vi "Get Result.vi"(6 "Last request":bool, 8 "error in (no error)":errorcluster, 11 "Temperature Controller Driver in":refnum<class "Temperature Controller Driver.lvclass">) -> (0 "error out":errorcluster, 2 "Result":refnum<class "Acquired Result.lvclass">, 3 "Temperature Controller Driver out":refnum<class "Temperature Controller Driver.lvclass">)   [LabVIEW 2024, in "Temperature Controller Driver.lvclass"]
uses:
  Temperature Controller Driver.lvclass
  Results/Acquired Result/Acquired Result.lvclass
  Temperature Controller Driver.lvclass/Temperature Controller Driver.ctl
  d4704567-7086-47cf-bd59-7ca7029b5dc6.vi
  28732cff-cc5e-42dd-a4af-5e59016cd5d7.vi
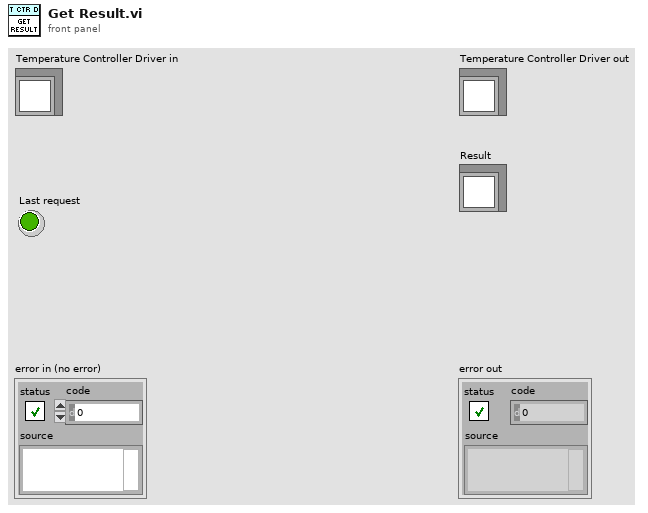
[diagram p1: front panel]
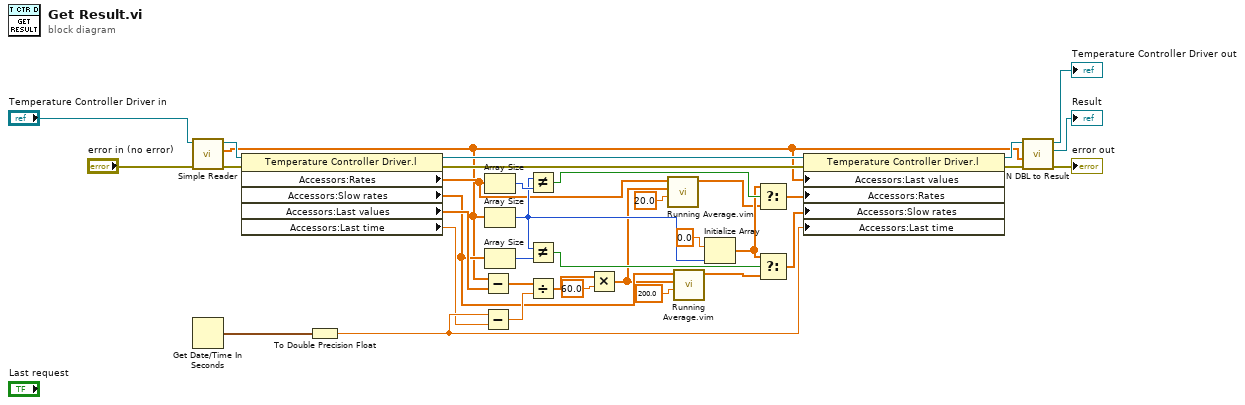
[diagram p0: block diagram]
diagram:
  n1 = call-dynamic "Simple Reader.vi"("error in (no error)"="error in (no error)", "Instrument Driver in"="Temperature Controller Driver in") -> ("error out"=w36:errorcluster, "Signals"=w4:dbl[], "Instrument Driver out"=w30:refnum<class "Temperature Controller Driver.lvclass">)  [unwired: 7 in]
  n2 = Get Date/Time In Seconds() -> (seconds since 1Jan1904=w23:timestamp)
  n3 = property class="Temperature Controller Driver.l"(reference=w30, error in=w36) -> (reference out=w28:refnum<class "Temperature Controller Driver.lvclass">, error out=w27:errorcluster, "Accessors:Rates"=w8:dbl[], "Accessors:Slow rates"=w5:dbl[], "Accessors:Last values"=w20:dbl[], "Accessors:Last time"=w21:dbl)
  n4 = To Double Precision Float(number=w23) -> (double precision float=w22:dbl)
  n5 = Subtract(x=w4, y=w20) -> (x-y=w19:dbl[])
  n6 = Subtract(x=w22, y=w21) -> (x-y=w18:dbl)
  n7 = Array Size(array=w8) -> (size(s)=w14:i32)
  n8 = Array Size(array=w4) -> (size(s)=w12:i32)
  n9 = Array Size(array=w5) -> (size(s)=w13:i32)
  n10 = Not Equal?(x=w12, y=w14) -> (x != y?=w29:bool)
  n11 = Not Equal?(x=w12, y=w13) -> (x != y?=w11:bool)
  n12 = Divide(x=w19, y=w18) -> (x/y=w17:dbl[])
  n13 = Multiply(x=w17, y=60.0) -> (x*y=w1:dbl[])
  n14 = call "Running Average.vim"("Averaging window"=20.0, "X"=w1, "Y"=w8) -> ("Y out"=w6:dbl[])  [unwired: 8 in]
  n15 = call "Running Average.vim"("Averaging window"=200.0, "X"=w1, "Y"=w5) -> ("Y out"=w2:dbl[])  [unwired: 8 in]
  n16 = Initialize Array(0.0 ("element"), w12) -> (w10:dbl[])
  n17 = Select(t=w10, s=w29, f=w6) -> (s? t:f=w24:dbl[])
  n18 = Select(t=w10, s=w11, f=w2) -> (s? t:f=w9:dbl[])
  n19 = property class="Temperature Controller Driver.l"(reference=w28, error in=w27, "Accessors:Last values"=w4, "Accessors:Rates"=w24, "Accessors:Slow rates"=w9, "Accessors:Last time"=w22) -> (reference out=w25:refnum<class "Temperature Controller Driver.lvclass">, error out=w26:errorcluster)
  n20 = call-dynamic "N DBL to Result.vi"("error in (no error)"=w26, "Data"=w4, "Instrument Driver in"=w25) -> ("error out"=→"error out":errorcluster, "Result out"=→"Result":refnum<class "Acquired Result.lvclass">, "Instrument Driver out"=→"Temperature Controller Driver out":refnum<class "Temperature Controller Driver.lvclass">)  [unwired: 6 in]
